vi "MICS, Telem Open Session.vi"(8 "error in":errorcluster, 9 "max attempts (1)":i32=1, 11 "VISA resource":refnum<visa-resource-name>="COM13") -> (0 "error out":errorcluster, 1 "in_session":bool, 3 "VISA resource dup":refnum<visa-resource-name>)   [LabVIEW 2020]
uses:
  Drivers/Telemetry/Typedef Command List.ctl
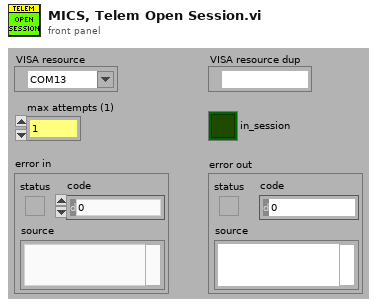
[diagram p1: front panel]
types:
  T1 = typedef "Typedef Command List.ctl" = enum16{"Get xPG Status", "xPG Stimulation", "Select Program", "Increment Program Amplitude", "Decrement Program Amplitude", "Get PoP Constants", "Get PPC Constants", "Get Program Names", "Set Pulse Amplitude", "Increment Pulse Amplitude", "Decrement Pulse Amplitude", "Get Pulse Widths", "Set Pulse Widths", "Increment Pulse Width", "Decrement Pulse Width", "Get Program Frequency", "Set Program Frequency", "Increment Program Frequency", "Decrement Program Frequency", "Inject Event", "Charging Control", "Get xPG Identity", "Set xPG Identity", "Restore Program Defaults", "Get Program Definition", "Set Program Definition", "Get Program Constants", "Set Program Constants", "Get Configurable Device Parameters", "Set Configurable Device Parameters", "Get Pulse Constants", "Set Pulse Constants", "Get Lead Limits", "Set Lead Limits", "Get Channel Calibrations", "Set Channel Calibrations", "<reserved 2>", "<reserved 3>", "<reserved 4>", "<reserved 5>", "<reserved 6>", "<reserved 7>", "Get Stim Asic HV Calibrations", "Set Stim Asic HV Calibrations", "<reserved 8>", "<reserved 9>", "Get CP Data", "Set CP Data", "Clear Log", "Read Log", "Append Log", "Get Patient Program Runtime", "Set Patient Program Runtime", "Impedance Measurement", "Enter Storage Mode", "Echo Short", "Echo Long", "Get General Calibration", "Set General Calibration", "Get Trim List", "Set Trim List", "Get Counter", "Set Counter", "Get Test Stimulation", "Set Test Stimulation", "Get Titration Stimulation", "Set Titration Stimulation", "Get Ramp Time", "Set Ramp Time", "Get VBAT", "Set Software Description Block", "Get Software Description Block", "Write Memory", "Read Memory", "Reset xPG", "Erase Flash Block", "Write Vectors", "Read Vectors", "Diagnostic Data", "Set Background Impedance", "Get Background Impedence ", "Set Test Waveform", "Calibrate Channel", "Get Log Range", "Reserved 0x55", "Reserved 0x56", "MICS Options", "Pair PPC", "Pair POP", "Stop Bootloader", "Tune MICS", "MICS Diagnostics", "Undefined"}
  T2 = cluster{"Command":T1, "Function":enum16{"Open Session", "Close Session", "Downlink Only", "Uplink Only", "Transceive (DN -> UP)"}, "MICS_ID":u32, "EXID":u32, "Use Local":bool, "Transceive Delay mS":dbl, "CP_DATA IN":u8[], "Parameters":string}
  T3 = cluster{"ERROR_OCCURRED":bool, "LINK_STAT_CHANGED":bool, "LINK_QUAL_CHANGED":bool, "400MHZ_TX_ACTIVE":bool, "400MHZ_RX_ACTIVE":bool, "245GHZ_TX_ACTIVE":bool, "DATA_STAT_CHANGED":bool, "SLEEPING":bool, "IDLE":bool, "SEARCHING_FOR_IMPLANT":bool, "STARTING_SESSION":bool, "LISTENING_FOR_EMERG":bool, "IN_SESSION":bool}
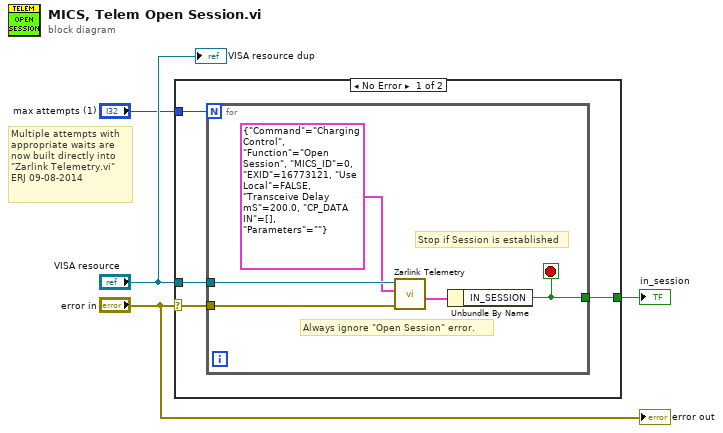
[diagram p0: block diagram]
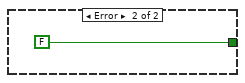
[diagram p2: hidden frame]
diagram:
  # "Multiple attempts with\nappropriate waits are\nnow built directly into\n\"Zarlink Telemetry.vi\"\nERJ 09-08-2014"
  n1 = case shown="No Error" "error in" {
    selector: "error in" -> [w6 _]
    tunnel: "VISA resource" -> [w8 _]
    tunnel: [w7 FALSE ("IN_SESSION")] -> w3
    tunnel: "max attempts (1)" -> [w5 _]
    frame No Error {
      n2 = for {
        N: w5 -> [_]
        tunnel: w8 -> [w13]
        tunnel: [w9] -> w7
        tunnel: w6 -> [w12]
        stop <- w9 stop-if-true
        # "Stop if Session is established"
        # "Always ignore \"Open Session\" error."
        n3 = call "Zarlink Telemetry.vi"("error in (no error)"=w12, "Input"=T2 {"Command"=enum."Charging Control", "Function"=enum."Open Session", "MICS_ID"=0, "EXID"=16773121, "Use Local"=FALSE, "Transceive Delay mS"=200.0, "CP_DATA IN"=[], "Parameters"=""}, "MICS Dongle Address"=w13) -> ("Status Flags"=w10:T3)  [unwired: 6 in, 2 out]
        n4 = Unbundle By Name(w10) -> ("IN_SESSION"=w9:bool)
      }
    }
    frame Error {
    }
  }
  "in_session" <- w3
  "error out" <- "error in"
  "VISA resource dup" <- "VISA resource"
